vi "niDAQmx Close gRPC Task.vi"(0 "task in":refnum<class "Session Factory.lvclass">, 11 "error in":errorcluster) -> (15 "error out":errorcluster)   [LabVIEW 2021, in "Session Management niDAQmx.lvlib" / "Session Factory.lvclass"]
doc: "Clears the niDAQmx task on the specified NI gRPC Device Server."
uses:
  Session Factory.lvclass
  NI DAQmx Client/RPC Messages/nidaqmx_grpc_ClearTaskRequest.ctl
  NI DAQmx Client/RPC Messages/nidevice_grpc_Session.ctl
  NI DAQmx Client/RPC Messages/nidevice_grpc_Session_session/nidevice_grpc_Session_session.lvclass
  Session Factory.lvclass/Session Factory.ctl
  NI DAQmx Client/NI_DAQmx_client.lvlib
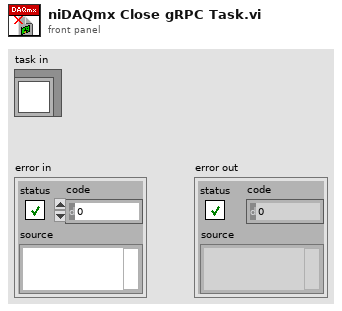
[diagram p1: front panel]
types:
  T1 = typedef "NI_DAQmx_client.lvlib/nidaqmx_grpc_ClearTaskRequest.ctl" = cluster{"task":T2}
  T2 = typedef "NI_DAQmx_client.lvlib/nidevice_grpc_Session.ctl" = cluster{"nidevice_grpc_Session_session":refnum<class "nidevice_grpc_Session_session.lvclass">}
  T3 = typedef "grpc-lvsupport-release.lvlib/grpcId.ctl" = u64
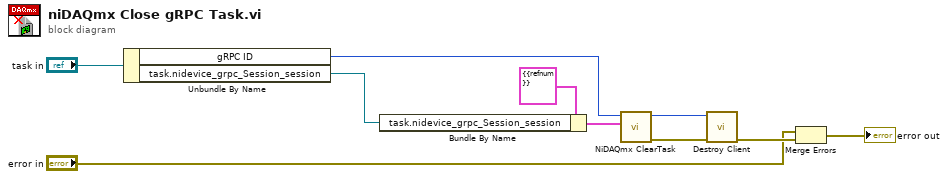
[diagram p0: block diagram]
diagram:
  n1 = Unbundle By Name("task in") -> ("gRPC ID"=w8:T3, "task.nidevice_grpc_Session_session"=w4:refnum<class "nidevice_grpc_Session_session.lvclass">)
  n2 = Bundle By Name(cluster=T1 {"task"={"nidevice_grpc_Session_session"=refnum}} ("Request Data"), "task.nidevice_grpc_Session_session"=w4) -> (w5:T1)
  n3 = call "NiDAQmx ClearTask.vi"("Request Data"=w5, "gRPC ID"=w8) -> ("error out"=w9:errorcluster, "gRPC ID out"=w7:T3)  [unwired: 7 in, 1 out]
  n4 = call "Destroy Client.vi"("error in"=w9, "gRPC ID"=w7) -> ("error out"=w3:errorcluster)  [unwired: 9 in]
  n5 = Merge Errors("error in", w3) -> (→"error out":errorcluster)
